vi "VISA02_ModbusRTU02_Write.vi"(11 "YTESTER测试数据":T1={"Socket(From1)"=1, "SN"=refnum, "StopFlagRef"=refnum, "YT System Queue"=refnum}) -> (3 "YTESTER结论":T2)   [LabVIEW 2017]
doc: "VIDescription=基于NI官方库的MODBUS操作"
uses:
  YtCommon.lvlibp/yt`Step StepBaseInput.ctl
  YtCommon.lvlibp/yt`Step StepResult.ctl
  YtCommon.lvlibp/yt`Step TestData.ctl
  YtCommon.lvlibp/yt`Step System Queue.ctl
  Step`s VIs/NI Modbus.llb/MB Serial Master Query Write Multiple Registers (poly).vi
  Step`s VIs/NI Modbus.llb/MB Serial Master Query Write Multiple Coils (poly).vi
  YtCommon.lvlibp
panel:
  in  "YTESTER开放参数":T4={"YTESTER_BaseInput"={"isTest"=FALSE, "isSkip"=FALSE, "StepName"="NI Modbus写", "OnPass"=enum."Next", "OnFail"=enum."Next", "ReTestNumber"=0.0}, "VISA resource"="", "baud rate (9600)"="9600", "Mode"=enum."RTU", "Slave Address"=1, "Timeout"=3000, "Starting Address"=0, "WriteType"=enum."Write Coils", "Coils"=[FALSE], "Registers"=[0]} {"Registers" format="%.0x"}
  # "Modbus\nWrite"
  # "Modbus四种数据类型：\n　　Discretes Input　　　　     位变量            只读\n　　Coils　　　　　　　　    　 位变量            读写\n　　Input Registers　　   　16-bit整型            只读\n　　Holding Registers 　    16-bit整型            读写"
  # "#yyll 采用NI-Modbus VI 内部存在耗时，待优化！！！"
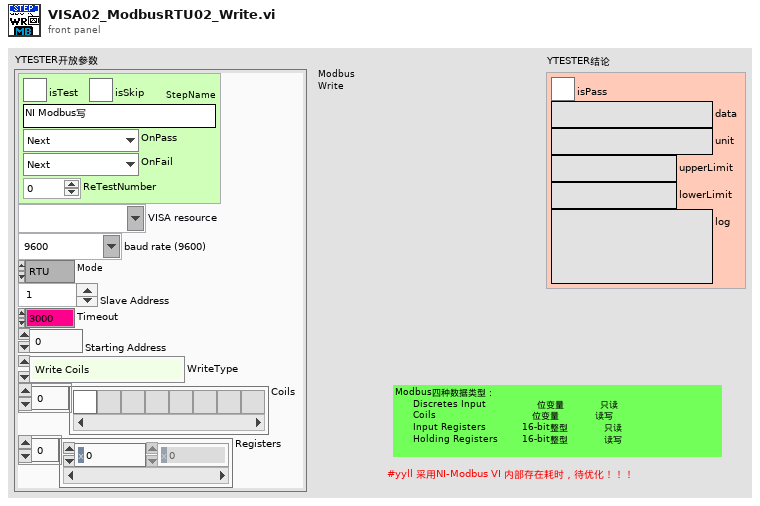
[diagram p1: front panel]
types:
  T1 = typedef "YtCommon.lvlibp/yt`Step TestData.ctl" = cluster{"Socket(From1)":i32, "SN":refnum<notifier>, "StopFlagRef":refnum<notifier>, "YT System Queue":refnum<queue>}
  T2 = typedef "YtCommon.lvlibp/yt`Step StepResult.ctl" = cluster{"isPass":bool, "data":string, "unit":string, "upperLimit":string, "lowerLimit":string, "log":string}
  T3 = typedef "YtCommon.lvlibp/yt`Step StepBaseInput.ctl" = cluster{"isTest":bool, "isSkip":bool, "StepName":string, "OnPass":enum16{"Next", "ToOVER", "Terminate"}, "OnFail":enum16{"Next", "ToOVER", "Terminate"}, "ReTestNumber":dbl}
  T4 = cluster{"YTESTER_BaseInput":T3, "VISA resource":refnum<visa-resource-name>, "baud rate (9600)":string, "Mode":enum16{"RTU", "ASCII"}, "Slave Address":u8, "Timeout":u32, "Starting Address":u16, "WriteType":enum16{"Write Coils", "Write Holding Registers"}, "Coils":bool[], "Registers":u16[]}
  T5 = cluster{"Mode":enum16{"RTU", "ASCII"}, "Slave Address":u8}
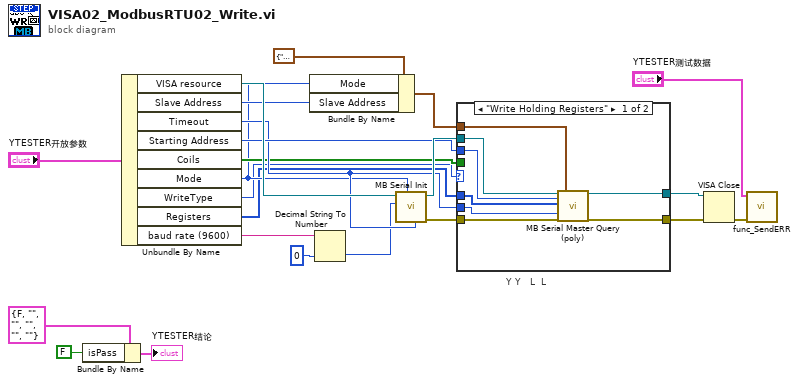
[diagram p0: block diagram]
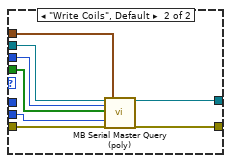
[diagram p2: hidden frame]
diagram:
  # "Y Y   L  L"
  n1 = Bundle By Name(cluster=T2 {"isPass"=FALSE, "data"="", "unit"="", "upperLimit"="", "lowerLimit"="", "log"=""} ("Result"), "isPass"=FALSE) -> (→"YTESTER结论":T2)
  n2 = Unbundle By Name("YTESTER开放参数") -> ("VISA resource"=w15:refnum<visa-resource-name>, "Slave Address"=w12:u8, "Timeout"=w10:u32, "Starting Address"=w11:u16, "Coils"=w7:bool[], "Mode"=w6:enum16{"RTU", "ASCII"}, "WriteType"=w5:enum16{"Write Coils", "Write Holding Registers"}, "Registers"=w4:u16[], "baud rate (9600)"=w2:string)
  n3 = Bundle By Name(cluster=T5 {"Mode"=enum."RTU", "Slave Address"=0} ("Serial Parameters"), "Mode"=w6, "Slave Address"=w12) -> (w13:T5)
  n4 = Decimal String To Number(string=w2, default (0L)=u32 0 ("default (0 I32)")) -> (number=w1:u32)  [unwired: 1 in, 1 out]
  n5 = call "MB Serial Init.vi"("Timeout"=w10, "Mode"=w6, "Baud Rate"=w1, "VISA resource name"=w15) -> ("error out"=w18:errorcluster, "VISA resource name out"=w20:refnum<visa-resource-name>)  [unwired: 3 in, 3 out]
  n6 = case shown="\"Write Holding Registers\"" w5 {
    tunnel: w20 -> [w31 w39]
    tunnel: [w30 w38] -> w19
    tunnel: w18 -> [w29 w37]
    tunnel: [w28 w36] -> w17
    tunnel: w13 -> [w27 w35]
    tunnel: w11 -> [w26 w34]
    tunnel: w10 -> [w25 w33]
    tunnel: w7 -> [_ w32]
    tunnel: w4 -> [w24 _]
    frame "Write Holding Registers" {
      n7 = call-poly "MB Serial Master Query (poly).vi"("VISA resource name"=w31, "Starting Address"=w26, "Registers"=w24, "Timeout"=w25, "error in"=w29, "Serial Parameters"=w27) -> ("VISA resource name out"=w30:refnum<visa-resource-name>, "error out"=w28:errorcluster)  [unwired: 12 out]
    }
    frame "Write Coils", Default {
      n8 = call-poly "MB Serial Master Query (poly).vi"("VISA resource name"=w39, "Starting Address"=w34, "Coils"=w32, "Timeout"=w33, "error in"=w37, "Serial Parameters"=w35) -> ("VISA resource name out"=w38:refnum<visa-resource-name>, "error out"=w36:errorcluster)  [unwired: 12 out]
    }
  }
  n9 = VISA Close(VISA resource name=w19, error in (no error)=w17) -> (error out=w9:errorcluster)
  n10 = call "func_SendERR.vi"("ERR (String\\Errclust)"=w9, "YTESTER测试数据 in"="YTESTER测试数据") -> ()  [unwired: 9 in, 1 out]
